vi "new edge detection.vi"(6 "rising edge (T)":bool=TRUE, 7 "switch encoders (F)":bool, 8 "ticks":u32[](array[numeric])=[0, 0], 9 "encoder 2":bool, 10 "encoder 1":bool, 11 "history in":bool[](array[boolean])=[FALSE, FALSE, FALSE, FALSE, FALSE, FALSE, FALSE, FALSE, FALSE, FALSE, FALSE, FALSE, FALSE, FALSE, FALSE, FALSE, FALSE, FALSE, FALSE, FALSE, FALSE, FALSE, FALSE, FALSE, FALSE, FALSE, FALSE, FALSE, FALSE, FALSE, FALSE, FALSE, FALSE, FALSE, FALSE, FALSE, FALSE, FALSE, FALSE, FALSE, FALSE, FALSE, FALSE, FALSE, FALSE, FALSE, FALSE, FALSE, FALSE, FALSE, FALSE, FALSE, FALSE, FALSE, FALSE, FALSE, FALSE, FALSE, FALSE, FALSE, FALSE, FALSE, FALSE, FALSE, FALSE, FALSE, FALSE, FALSE, FALSE, FALSE, FALSE, FALSE, FALSE, FALSE, FALSE, FALSE, FALSE, FALSE, FALSE, FALSE, FALSE, FALSE, FALSE, FALSE, FALSE, FALSE, FALSE, FALSE, FALSE, FALSE, FALSE, FALSE, FALSE, FALSE, FALSE, FALSE, FALSE, FALSE, FALSE, FALSE]) -> (0 "ticks out":u32[](array[numeric]), 1 "edge detected":bool, 3 "history out":bool[](array[boolean]))   [LabVIEW 2018]
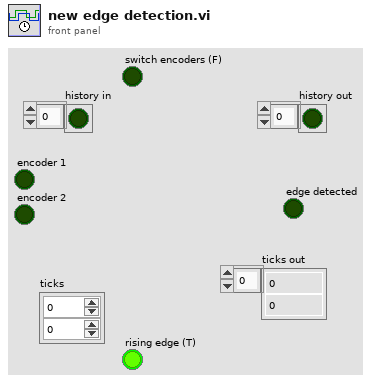
[diagram p1: front panel]
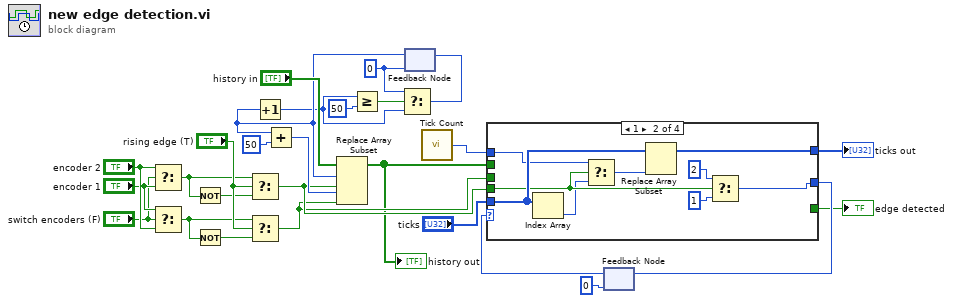
[diagram p0: block diagram]
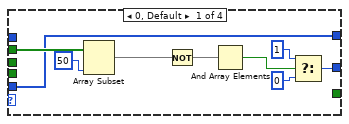
[diagram p2: hidden frame]
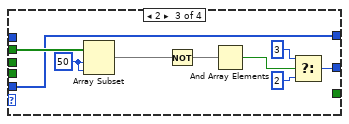
[diagram p3: hidden frame]
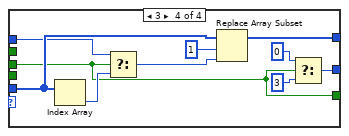
[diagram p4: hidden frame]
diagram:
  w18 = i16 0 ("t")
  n1 = Select(t="encoder 2", s="switch encoders (F)", f="encoder 1") -> (s? t:f=w3:bool)
  n2 = Select(t="encoder 1", s="switch encoders (F)", f="encoder 2") -> (s? t:f=w2:bool)
  n3 = Not(x=w3) -> (.not. x?=w23:bool)
  n4 = Not(x=w2) -> (.not. x?=w22:bool)
  n5 = Select(t=w3, s="rising edge (T)", f=w23) -> (s? t:f=w13:bool)
  n6 = Select(t=w2, s="rising edge (T)", f=w22) -> (s? t:f=w12:bool)
  n7 = feedback #1(w18) -> (w19:i16)
  n8 = Increment(x=w19) -> (x+1=w16:i16)
  n9 = Add(x=w19, y=i16 50) -> (x+y=w27:i16)
  n10 = Replace Array Subset(array="history in", new element #1=w13, index #1=w19, new element #2=w12, index #2=w27) -> (w11:bool[])
  "history out" <- w11
  n11 = Greater Or Equal?(x=w16, y=i16 50 ("x")) -> (x >= y?=w25:bool)
  n12 = Select(t=w18, s=w25, f=w16) -> (s? t:f=w20:i16)
  n13 = feedback-in #1(w20) -> ()
  n14 = call "Tick Count"() -> ("Tick Count(Ticks)"=w1:u32)
  n15 = feedback #2(u8 0 ("f")) -> (w8:u8)
  n16 = case shown="1" w8 {
    tunnel: w11 -> [w33 _ w51 _]
    tunnel: [w30 w44 w47 w63] -> w9
    tunnel: w13 -> [_ w41 _ _]
    tunnel: w12 -> [_ _ _ w55]
    tunnel: "ticks" -> [w28 w43 w46 w60]
    tunnel: [w28 w42 w46 w61] -> w10
    tunnel: w1 -> [_ w40 _ w57]
    tunnel: [_ _ _ w55] -> w7
    frame 0, Default {
      n17 = Array Subset(array=w33, length=50) -> (w36:bool[])  [unwired: 1 in]
      n18 = Not(x=w36) -> (.not. x?=w35:bool[])
      n19 = And Array Elements(Boolean array=w35) -> (logical AND=w32:bool)
      n20 = Select(t=u8 1 ("next state"), s=w32, f=u8 0 ("next state")) -> (s? t:f=w30:u8)
    }
    frame 1 {
      n21 = Index Array(array=w43) -> (element=w39:u32)  [unwired: 1 in]
      n22 = Select(t=w40, s=w41, f=w39) -> (s? t:f=w38:u32)
      n23 = Replace Array Subset(array=w43, new element=w38) -> (w42:u32[])  [unwired: 1 in]
      n24 = Select(t=u8 2, s=w41, f=u8 1) -> (s? t:f=w44:u8)
    }
    frame 2 {
      w52 = 50 ("length")
      n25 = Array Subset(array=w51, index=w52, length=w52) -> (w54:bool[])
      n26 = Not(x=w54) -> (.not. x?=w53:bool[])
      n27 = And Array Elements(Boolean array=w53) -> (logical AND=w48:bool)
      n28 = Select(t=u8 3, s=w48, f=u8 2) -> (s? t:f=w47:u8)
    }
    frame 3 {
      n29 = Index Array(array=w60) -> (element=w59:u32)  [unwired: 1 in]
      n30 = Select(t=w57, s=w55, f=w59) -> (s? t:f=w58:u32)
      n31 = Replace Array Subset(array=w60, new element=w58, index=1) -> (w61:u32[])
      n32 = Select(t=u8 0, s=w55, f=u8 3) -> (s? t:f=w63:u8)
    }
  }
  "edge detected" <- w7
  "ticks out" <- w10
  n33 = feedback-in #2(w9) -> ()
